vi "side_giltch_damaged_detector.vi"(10 "D of clusters":cluster{"D":ext[]}[](array[cluster]), 11 "side of clusters":cluster{"Array out":dbl[][]}[](array[cluster])) -> (0 "damaged clusters":cluster{"damaged coord":dbl[]}[](array[cluster]), 1 "giltch of clusters":cluster{"giltch_coord":dbl[]}[](array[cluster]), 2 "D damaged of clusters":cluster{"D_damaged":ext}[](array[cluster]), 3 "D giltch of clusters":cluster{"D_giltch":ext}[](array[cluster]))   [LabVIEW 2017]
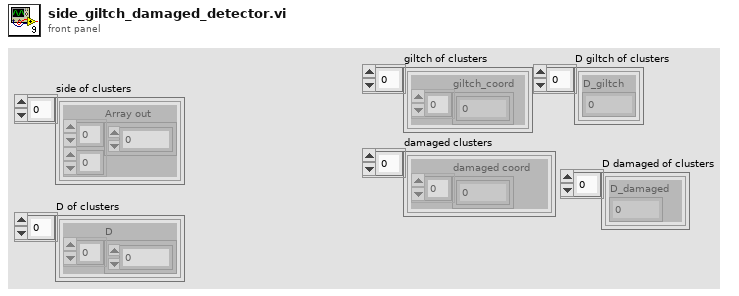
[diagram p1: front panel]
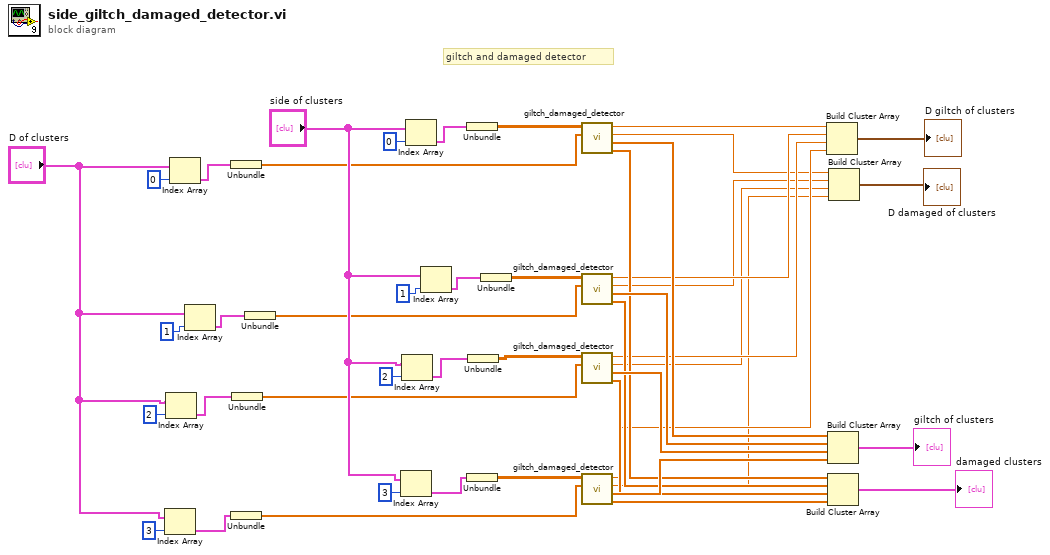
[diagram p0: block diagram]
diagram:
  # "giltch and damaged detector"
  n1 = Index Array(array="D of clusters", index=3 ("index (page)")) -> (element=w26:cluster{"D":ext[]})
  n2 = Index Array(array="D of clusters", index=2 ("index (page)")) -> (element=w27:cluster{"D":ext[]})
  n3 = Index Array(array="D of clusters", index=0 ("index (page)")) -> (element=w29:cluster{"D":ext[]})
  n4 = Index Array(array="D of clusters", index=1 ("index (page)")) -> (element=w28:cluster{"D":ext[]})
  n5 = Unbundle(w29) -> ("D"=w24:ext[])
  n6 = Unbundle(w26) -> ("D"=w21:ext[])
  n7 = Unbundle(w27) -> ("D"=w22:ext[])
  n8 = Unbundle(w28) -> ("D"=w23:ext[])
  n9 = Index Array(array="side of clusters", index=3 ("index (page)")) -> (element=w46:cluster{"Array out":dbl[][]})
  n10 = Index Array(array="side of clusters", index=2 ("index (page)")) -> (element=w45:cluster{"Array out":dbl[][]})
  n11 = Index Array(array="side of clusters", index=0 ("index (page)")) -> (element=w43:cluster{"Array out":dbl[][]})
  n12 = Index Array(array="side of clusters", index=1 ("index (page)")) -> (element=w44:cluster{"Array out":dbl[][]})
  n13 = Unbundle(w43) -> ("Array out"=w37:dbl[][])
  n14 = Unbundle(w46) -> ("Array out"=w34:dbl[][])
  n15 = Unbundle(w45) -> ("Array out"=w35:dbl[][])
  n16 = Unbundle(w44) -> ("Array out"=w36:dbl[][])
  n17 = call "giltch_damaged_detector.vi"("D"=w24, "side points"=w37) -> ("damaged coord"=w13:dbl[], "giltch_coord"=w20:dbl[], "D_damaged"=w5:ext, "D_giltch"=w10:ext)  [unwired: 6 in]
  n18 = call "giltch_damaged_detector.vi"("D"=w23, "side points"=w36) -> ("damaged coord"=w14:dbl[], "giltch_coord"=w19:dbl[], "D_damaged"=w4:ext, "D_giltch"=w9:ext)  [unwired: 6 in]
  n19 = call "giltch_damaged_detector.vi"("D"=w22, "side points"=w35) -> ("damaged coord"=w15:dbl[], "giltch_coord"=w18:dbl[], "D_damaged"=w3:ext, "D_giltch"=w8:ext)  [unwired: 6 in]
  n20 = call "giltch_damaged_detector.vi"("D"=w21, "side points"=w34) -> ("damaged coord"=w16:dbl[], "giltch_coord"=w17:dbl[], "D_damaged"=w2:ext, "D_giltch"=w7:ext)  [unwired: 6 in]
  n21 = Build Cluster Array(w10, w9, w8, w7) -> (→"D giltch of clusters":cluster{"D_giltch":ext}[])
  n22 = Build Cluster Array(w20, w19, w18, w17) -> (→"giltch of clusters":cluster{"giltch_coord":dbl[]}[])
  n23 = Build Cluster Array(w13, w14, w15, w16) -> (→"damaged clusters":cluster{"damaged coord":dbl[]}[])
  n24 = Build Cluster Array(w5, w4, w3, w2) -> (→"D damaged of clusters":cluster{"D_damaged":ext}[])
